vi "Check if Executable program.vi"() -> (0 "Exe?":bool)   [LabVIEW 2019]
doc: "Revision: 11.05.97\nDescription: Exit program if it is an executable\nGlobals: None\nWrite:None\nOccurrences: none\nDevices: none\nFiles: none\nSystem: none"
panel:
  out "error out":errorcluster
  in  "error in (no error)":errorcluster
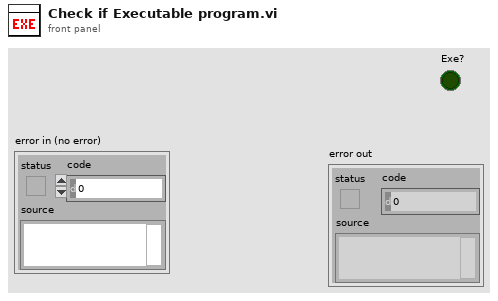
[diagram p1: front panel]
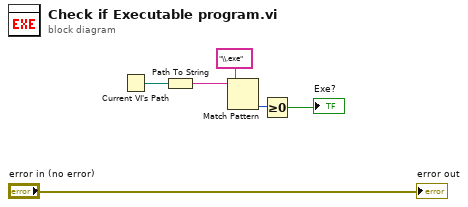
[diagram p0: block diagram]
diagram:
  n1 = Current VI's Path() -> (path=w2:path)
  n2 = Path To String(path=w2) -> (string=w1:string)
  n3 = Match Pattern(string=w1, regular expression="\\.exe") -> (offset past match=w5:i32)  [unwired: 1 in, 3 out]
  n4 = Greater Or Equal To 0?(x=w5) -> (x >= 0?=→"Exe?":bool)
  "error out" <- "error in (no error)"
